vi "subVI-Puertas.vi"(2 "Abrir":bool, 3 "Cerrar":bool, 4 "Bajar":bool, 5 "Subir":bool, 6 "Sensor-Obstruccion":bool, 7 "Sensor-Piso":bool) -> (0 "P-der":dbl(slide) scale=0.0..10.0, 1 "P-izq":dbl(slide))   [LabVIEW 2018]
panel:
  out "TIEMPO (SEG)":dbl
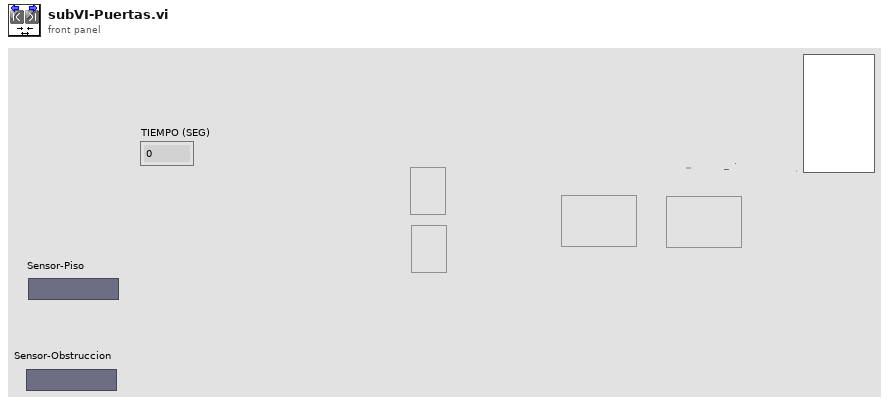
[diagram p1: front panel]
types:
  T1 = enum16{"estado-reposo", "estado-abrir", "temporizar", "Estado-cerrar", "estado-terminar"}
  T2 = enum8{"Enabled", "Disabled", "Disabled and Grayed Out"}
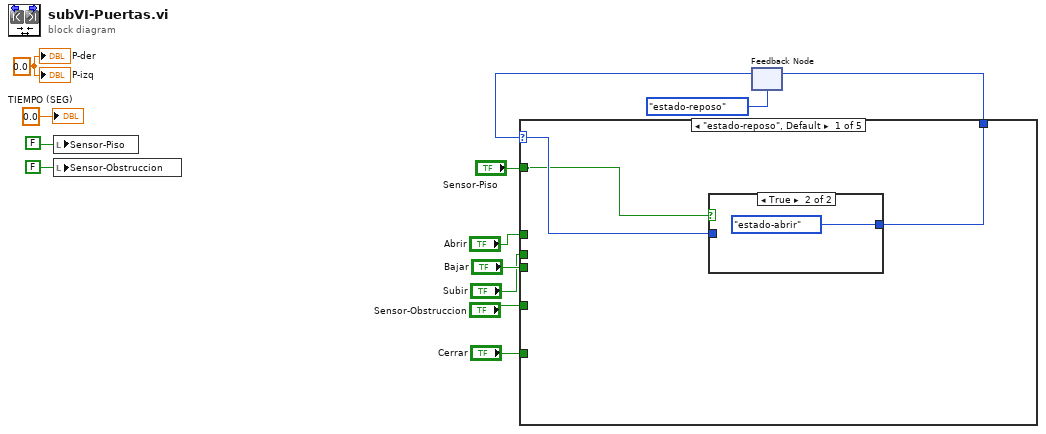
[diagram p0: block diagram]
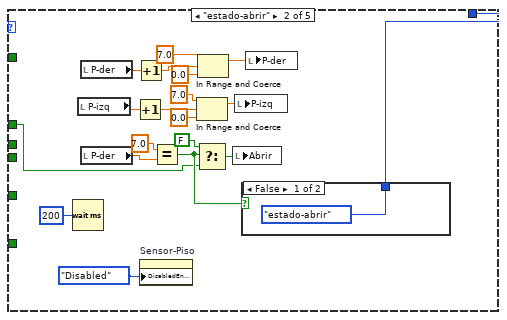
[diagram p3: hidden frame]
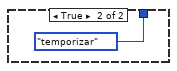
[diagram p4: hidden frame]
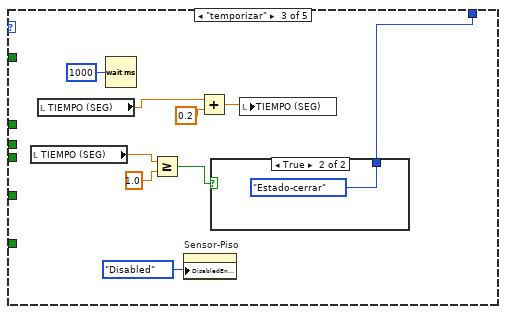
[diagram p5: hidden frame]
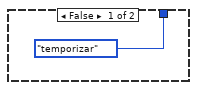
[diagram p6: hidden frame]
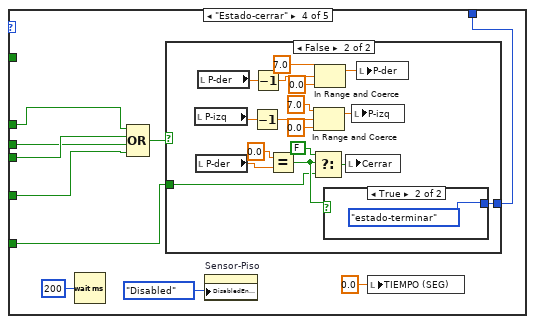
[diagram p7: hidden frame]
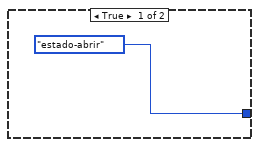
[diagram p8: hidden frame]
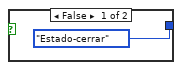
[diagram p9: hidden frame]
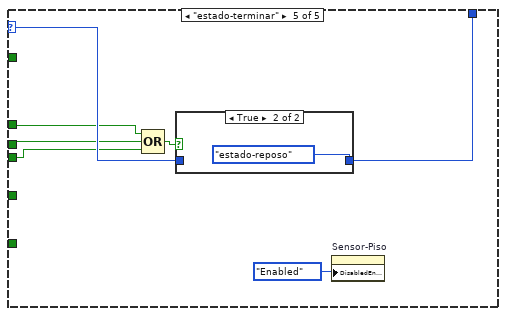
[diagram p10: hidden frame]
diagram:
  w11 = 0.0 ("P-izq")
  n1 = local write "Sensor-Piso"(FALSE ("Sensor-Piso")) -> ()
  n2 = local write "Sensor-Obstruccion"(FALSE ("Sensor-Piso")) -> ()
  n3 = feedback #1(T1."estado-reposo") -> (w8:T1)
  n4 = case shown="\"estado-reposo\", Default" w8 {
    selector: w8 -> [w15 _ _ _ w85]
    tunnel: [w16 w21 w46 w59 w86] -> w7
    tunnel: "Sensor-Piso" -> [w14 _ _ _ _]
    tunnel: "Abrir" -> [_ w19 _ w55 w83]
    tunnel: "Bajar" -> [_ _ _ w54 w82]
    tunnel: "Subir" -> [_ _ _ w53 w81]
    tunnel: "Sensor-Obstruccion" -> [_ _ _ w52 _]
    tunnel: "Cerrar" -> [_ _ _ w51 _]
    frame "estado-reposo", Default {
      n5 = case shown="True" w14 {
        tunnel: [w17 T1."estado-abrir"] -> w16
        tunnel: w15 -> [w17 _]
        frame False {
        }
        frame True {
        }
      }
    }
    frame "estado-abrir" {
      n6 = Wait (ms)(milliseconds to wait=u32 200) -> ()  [unwired: 1 out]
      n7 = local read "P-izq"() -> (w31:dbl)
      n8 = local read "P-der"() -> (w32:dbl)
      n9 = local read "P-der"() -> (w37:dbl)
      n10 = Increment(x=w31) -> (x+1=w35:dbl)
      n11 = Increment(x=w32) -> (x+1=w33:dbl)
      n12 = property on="Sensor-Piso" class="Bool (strict)"("DisabledEnum"=T2."Disabled" ("Disabled")) -> ()  [unwired: 2 in, 2 out]
      n13 = Equal?(x=7.0, y=w37) -> (x = y?=w30:bool)
      n14 = In Range and Coerce(upper limit=7.0, x=w35, lower limit=0.0) -> (coerced(x)=w34:dbl)  [unwired: 1 out]
      n15 = Select(t=FALSE ("Abrir"), s=w30, f=w19) -> (s? t:f=w36:bool)
      n16 = In Range and Coerce(upper limit=7.0, x=w33, lower limit=0.0) -> (coerced(x)=w20:dbl)  [unwired: 1 out]
      n17 = local write "Abrir"(w36) -> ()
      n18 = local write "P-izq"(w34) -> ()
      n19 = case shown="False" w30 {
        tunnel: [T1."estado-abrir" T1."temporizar"] -> w21
        frame False {
        }
        frame True {
        }
      }
      n20 = local write "P-der"(w20) -> ()
    }
    frame "temporizar" {
      n21 = local read "TIEMPO (SEG)"() -> (w41:dbl)
      n22 = local read "TIEMPO (SEG)"() -> (w42:dbl)
      n23 = Wait (ms)(milliseconds to wait=u32 1000) -> ()  [unwired: 1 out]
      n24 = Greater Or Equal?(x=w41, y=1.0) -> (x >= y?=w40:bool)
      n25 = property on="Sensor-Piso" class="Bool (strict)"("DisabledEnum"=T2."Disabled" ("Disabled")) -> ()  [unwired: 2 in, 2 out]
      n26 = Add(x=w42, y=0.2) -> (x+y=w44:dbl)
      n27 = case shown="True" w40 {
        tunnel: [T1."temporizar" T1."Estado-cerrar"] -> w46
        frame False {
        }
        frame True {
        }
      }
      n28 = local write "TIEMPO (SEG)"(w44) -> ()
    }
    frame "Estado-cerrar" {
      n29 = Wait (ms)(milliseconds to wait=u32 200) -> ()  [unwired: 1 out]
      n30 = Compound Arithmetic op=OR(w55, w54, w53, w52) -> (w56:bool)
      n31 = case shown="False" w56 {
        tunnel: [T1."estado-abrir" w63] -> w59
        tunnel: w51 -> [_ w62]
        frame True {
        }
        frame False {
          n32 = local read "P-izq"() -> (w78:dbl)
          n33 = local read "P-der"() -> (w71:dbl)
          n34 = local read "P-der"() -> (w77:dbl)
          n35 = Decrement(x=w78) -> (x-1=w73:dbl)
          n36 = Decrement(x=w77) -> (x-1=w76:dbl)
          n37 = Equal?(x=0.0, y=w71) -> (x = y?=w70:bool)
          n38 = Select(t=FALSE ("Abrir"), s=w70, f=w62) -> (s? t:f=w72:bool)
          n39 = In Range and Coerce(upper limit=7.0, x=w73, lower limit=0.0) -> (coerced(x)=w74:dbl)  [unwired: 1 out]
          n40 = In Range and Coerce(upper limit=7.0, x=w76, lower limit=0.0) -> (coerced(x)=w75:dbl)  [unwired: 1 out]
          n41 = case shown="True" w70 {
            tunnel: [T1."Estado-cerrar" T1."estado-terminar"] -> w63
            frame False {
            }
            frame True {
            }
          }
          n42 = local write "Cerrar"(w72) -> ()
          n43 = local write "P-izq"(w74) -> ()
          n44 = local write "P-der"(w75) -> ()
        }
      }
      n45 = property on="Sensor-Piso" class="Bool (strict)"("DisabledEnum"=T2."Disabled" ("Disabled")) -> ()  [unwired: 2 in, 2 out]
      n46 = local write "TIEMPO (SEG)"(0.0 ("TIEMPO (SEG)")) -> ()
    }
    frame "estado-terminar" {
      n47 = Compound Arithmetic op=OR(w83, w81, w82) -> (w84:bool)
      n48 = case shown="True" w84 {
        tunnel: [w88 T1."estado-reposo"] -> w86
        tunnel: w85 -> [w88 _]
        frame False {
        }
        frame True {
        }
      }
      n49 = property on="Sensor-Piso" class="Bool (strict)"("DisabledEnum"=T2."Enabled" ("Disabled")) -> ()  [unwired: 2 in, 2 out]
    }
  }
  n50 = feedback-in #1(w7) -> ()
  "P-izq" <- w11
  "P-der" <- w11
  "TIEMPO (SEG)" <- 0.0 ("TIEMPO (SEG)")
